vi "Init Events.vi"(8 "error in (no error)":errorcluster, 11 "Historian Charting Manager in":refnum<class "Historian Charting Manager.lvclass">) -> (0 "error out":errorcluster, 3 "Historian Charting Manager out":refnum<class "Historian Charting Manager.lvclass">)   [LabVIEW 2020, in "VolatusGUI.lvlib" / "Historian Charting Manager.lvclass"]
uses:
  Historian Charting Manager.lvclass
  Historian Charting Manager.lvclass/Historian Charting Manager.ctl
  New Plot Group Data.ctl
  X-Axis Type.ctl
  Scale.ctl
  Plot Config.ctl
  Plot Group Config.ctl
  Plot Group Changed Data.ctl
  Plot Group Removed Data.ctl
  Chart Select Group Data.ctl
  Plot Group Events.ctl
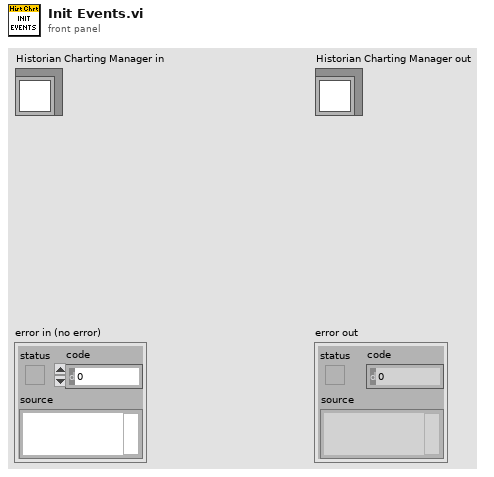
[diagram p1: front panel]
types:
  T1 = typedef "VolatusGUI.lvlib/Historian Charting Manager.lvclass/Plot Group Removed Data.ctl" = cluster{"Name":string, "Plot Groups":string[]}
  T2 = typedef "VolatusGUI.lvlib/Historian Charting Manager.lvclass/Plot Group Events.ctl" = cluster{"Changed":refnum<user-event>, "Removed":refnum<user-event>, "New":refnum<user-event>, "Select":refnum<user-event>}
  T3 = typedef "VolatusGUI.lvlib/Historian Charting Manager.lvclass/Plot Group Changed Data.ctl" = cluster{"Config":T4}
  T4 = typedef "VolatusGUI.lvlib/Historian Charting Manager.lvclass/Plot Group Config.ctl" = cluster{"Name":string, "X-Axis Type":T5, "X-Axis Channel":string, "Plots":T6[], "Lock Now":bool, "Time":string, "Swap Axes":bool}
  T5 = typedef "VolatusGUI.lvlib/Historian Charting Manager.lvclass/X-Axis Type.ctl" = enum16{"Time", "Channel"}
  T6 = typedef "VolatusGUI.lvlib/Historian Charting Manager.lvclass/Plot Config.ctl" = cluster{"Channel":string, "Visible":bool, "Color":u32, "Scale":T7}
  T7 = typedef "VolatusGUI.lvlib/Historian Charting Manager.lvclass/Scale.ctl" = enum16{"Left", "Right"}
  T8 = typedef "VolatusGUI.lvlib/Historian Charting Manager.lvclass/New Plot Group Data.ctl" = cluster{"Name":string, "Plot Groups":string[]}
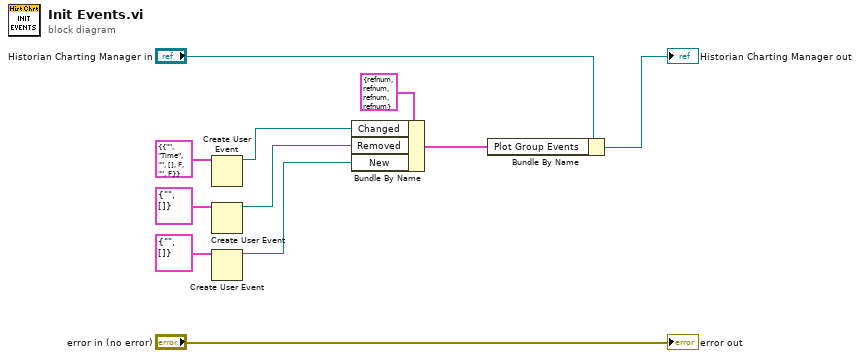
[diagram p0: block diagram]
diagram:
  n1 = Create User Event(user event datatype=T3 {"Config"={"Name"="", "X-Axis Type"=enum."Time", "X-Axis Channel"="", "Plots"=[], "Lock Now"=FALSE, "Time"="", "Swap Axes"=FALSE}} ("Plot Group Changed Data")) -> (user event=w6:refnum<user-event>)  [unwired: 1 in, 1 out]
  n2 = Create User Event(user event datatype=T1 {"Name"="", "Plot Groups"=[]} ("Plot Group Removed Data")) -> (user event=w4:refnum<user-event>)  [unwired: 1 in, 1 out]
  n3 = Create User Event(user event datatype=T8 {"Name"="", "Plot Groups"=[]} ("New Plot Group Data")) -> (user event=w3:refnum<user-event>)  [unwired: 1 in, 1 out]
  n4 = Bundle By Name(cluster=T2 {"Changed"=refnum, "Removed"=refnum, "New"=refnum, "Select"=refnum} ("Plot Group Events"), "Changed"=w6, "Removed"=w4, "New"=w3) -> (w1:T2)
  n5 = Bundle By Name(cluster="Historian Charting Manager in", "Plot Group Events"=w1) -> (→"Historian Charting Manager out":refnum<class "Historian Charting Manager.lvclass">)
  "error out" <- "error in (no error)"
